vi "Actor.vi"(0 "Path":path, 4 "Creator":refnum<user-event>, 6 "Creator Alias":string, 8 "Self Alias":string, 9 "Queue of Created Info":refnum<queue>, 10 "Actor":refnum<class "Actor.lvclass">) -> ()   [LabVIEW 2021, in "jettl.lvlib" / "Actor.lvlib" / "Base Actor.lvclass"]
uses:
  Base Actor.lvclass
  Actor/Actor.lvclass
  Msg/Msg.lvclass
  Created Info/Created Info.lvclass
  C:/git/jettl/jettl/jettl/Actor/Actor/Actor.lvclass
  Base Actor.lvclass/Base Actor.ctl
  Addresses Strategy/Addresses Strategy.lvlib
  Last Ack Msg/Last Ack Msg.lvlib
  C:/git/jettl/jettl/jettl/Last Ack Msg/Last Ack/Last Ack.lvclass
  C:/git/jettl/jettl/jettl/Setup Msg/Setup/Setup.lvclass
  C:/git/jettl/jettl/jettl/Teardown Msg/Teardown/Teardown.lvclass
  Actor.lvlib
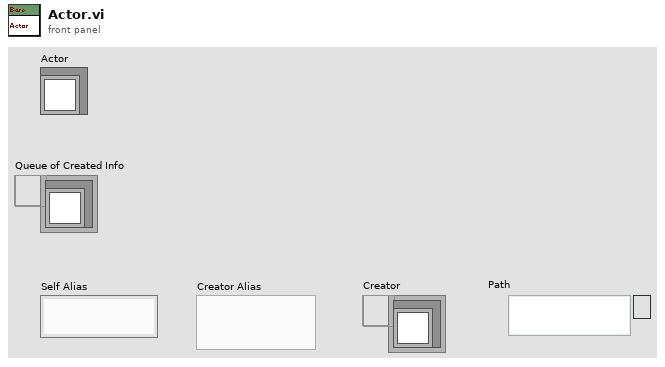
[diagram p1: front panel]
types:
  T1 = typedef "jettl.lvlib/Utilities.lvlib/Set of Msgs.ctl" = set{refnum<class "Msg.lvclass">}
  T2 = typedef "jettl.lvlib/Utilities.lvlib/Created Aliases.ctl" = set{string}
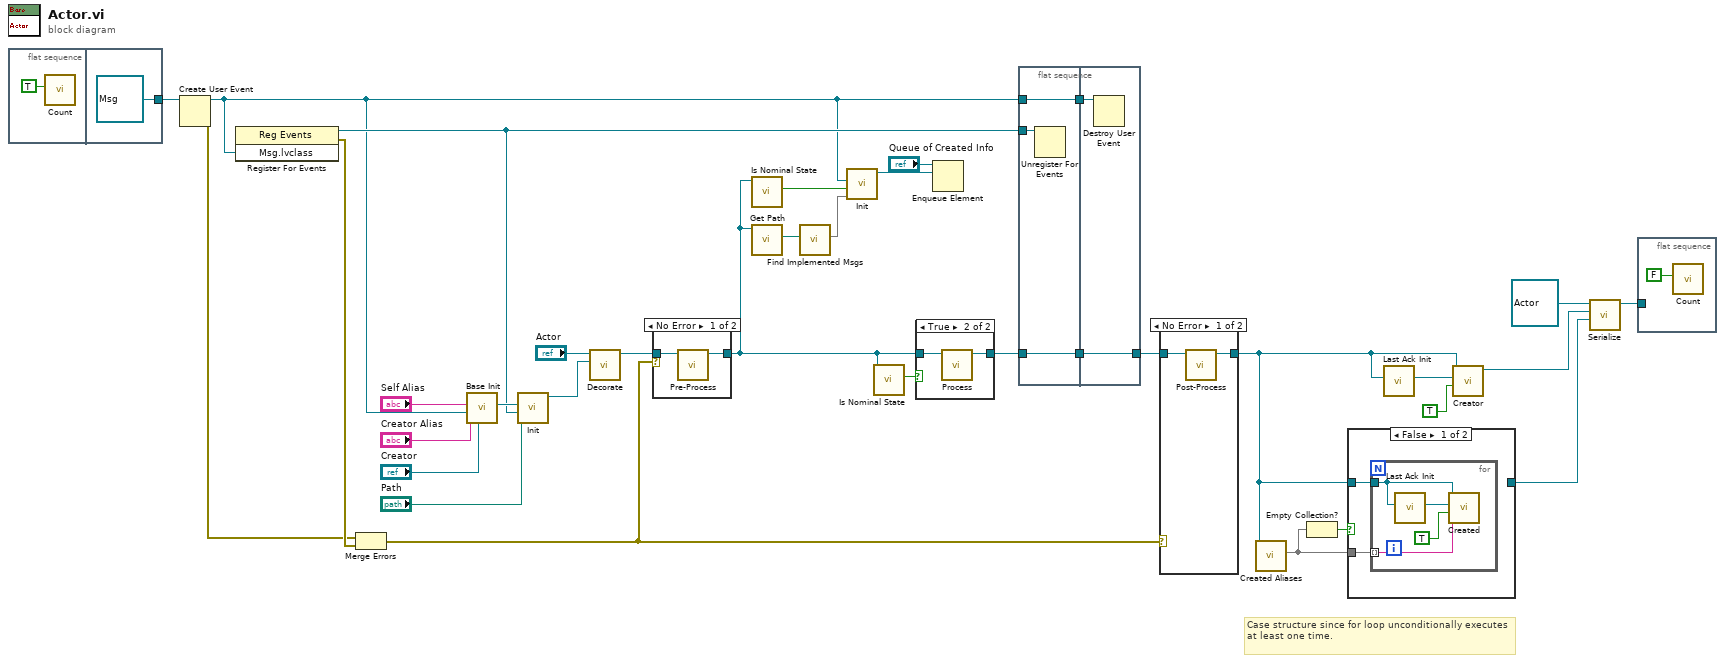
[diagram p0: block diagram]
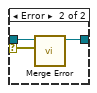
[diagram p2: hidden frame]
diagram:
  # "Case structure since for loop unconditionally executes at least one time."
  n1 = flat-sequence {
    tunnel: [refnum<class "Msg.lvclass"> refnum ("Msg.lvclass")] -> w28
    frame #0 {
      n2 = call "Count.vi"("Increment?"=TRUE) -> ()  [unwired: 11 in]
    }
    frame #1 {
    }
  }
  n3 = Create User Event(user event datatype=w28) -> (user event=w6:refnum<user-event>, error out=w30:errorcluster)  [unwired: 1 in]
  n4 = register-events(w6) -> (reference out=w21:refnum<event-registration>, error out=w32:errorcluster)  [unwired: 2 in]
  n5 = Merge Errors(w30, w32) -> (w18:errorcluster)
  n6 = call "Base Init.vi"("Creator"="Creator", "Creator Alias"="Creator Alias", "Self"=w6, "Self Alias"="Self Alias") -> ("Addresses Strategy out"=w29:refnum<class "Addresses Strategy.lvclass">)  [unwired: 7 in]
  n7 = call "Init.vi"("Path"="Path", "Register"=w21, "Addresses Strategy"=w29) -> ("Base Actor out"=w26:refnum<class "Base Actor.lvclass">)  [unwired: 8 in]
  n8 = call-dynamic "Decorate.vi"("Actor"=w26, "Actor in"="Actor") -> ("Actor out"=w25:refnum<class "Actor.lvclass">)  [unwired: 9 in]
  n9 = case shown="No Error" w18 {
    selector: w18 -> [_ w39]
    tunnel: [w38 w40] -> w3
    tunnel: w25 -> [w37 w41]
    frame No Error {
      n10 = call-dynamic "Pre-Process.vi"("Actor in"=w37) -> ("Actor out"=w38:refnum<class "Actor.lvclass">)  [unwired: 10 in]
    }
    frame Error {
      n11 = call-dynamic "Merge Error.vi"("Error"=w39, "Actor in"=w41) -> ("Actor out"=w40:refnum<class "Actor.lvclass">)  [unwired: 9 in]
    }
  }
  n12 = call-dynamic "Is Nominal State.vi"("Actor in"=w3) -> ("Is Nominal State?"=w2:bool)  [unwired: 10 in]
  n13 = call-dynamic "Get Path.vi"("Actor in"=w3) -> ("Path"=w4:path)  [unwired: 10 in]
  n14 = call "Find Implemented Msgs.vi"("Path"=w4) -> ("Set of Msgs"=w5:T1)  [unwired: 10 in]
  n15 = call "Init.vi"("Set of Msgs"=w5, "Is Normal"=w2, "Self"=w6) -> ("Created Info out"=w7:refnum<class "Created Info.lvclass">)  [unwired: 8 in]
  n16 = call-dynamic "Is Nominal State.vi"("Actor in"=w3) -> ("Is Nominal State?"=w1:bool)  [unwired: 10 in]
  n17 = case shown="True" w1 {
    tunnel: w3 -> [w42 w44]
    tunnel: [w42 w43] -> w22
    frame False {
    }
    frame True {
      n18 = call-dynamic "Process.vi"("Actor in"=w44) -> ("Actor out"=w43:refnum<class "Actor.lvclass">)  [unwired: 10 in]
    }
  }
  n19 = Enqueue Element(queue="Queue of Created Info", element=w7) -> ()  [unwired: 2 in, 3 out]
  n20 = flat-sequence {
    tunnel: [w47] -> w23
    tunnel: w22 -> [w47]
    tunnel: w21 -> [w46]
    tunnel: w6 -> [w45]
    tunnel: [w45] -> w20
    tunnel: [w49] -> w24
    tunnel: w23 -> [w49]
    tunnel: w20 -> [w48]
    frame #0 {
      n21 = Unregister For Events(event registration refnum=w46) -> ()  [unwired: 1 in, 1 out]
    }
    frame #1 {
      n22 = Destroy User Event(user event=w48) -> ()  [unwired: 1 in, 1 out]
    }
  }
  n23 = case shown="No Error" w18 {
    tunnel: w24 -> [w51 w52]
    tunnel: [w50 w52] -> w12
    frame No Error {
      n24 = call-dynamic "Post-Process.vi"("Actor in"=w51) -> ("Actor out"=w50:refnum<class "Actor.lvclass">)  [unwired: 10 in]
    }
    frame Error {
    }
  }
  n25 = call-dynamic "Created Aliases.vi"("Actor in"=w12) -> ("Created Aliases"=w14:T2)  [unwired: 10 in]
  n26 = Empty Collection?(1:w14) -> (0:w15:bool)
  n27 = case shown="False" w15 {
    tunnel: w14 -> [w54 _]
    tunnel: w12 -> [w53 w59]
    tunnel: [_ w59] -> w10
    frame False {
      n28 = for {
        tunnel: w53 -> [w56]
        tunnel: w54 -> [w58] mode=indexing
        n29 = call "Last Ack Init.vi"("Actor"=w56) -> ("Msg"=w55:refnum<class "Msg.lvclass">)  [unwired: 10 in]
        n30 = call-dynamic "Created.vi"("Created Alias"=w58, "Is Priority"=TRUE ("Priority?"), "Msg"=w55, "Actor in"=w56) -> ()  [unwired: 7 in, 1 out]
      }
    }
    frame True {
    }
  }
  n31 = call "Last Ack Init.vi"("Actor"=w12) -> ("Msg"=w16:refnum<class "Msg.lvclass">)  [unwired: 10 in]
  n32 = call-dynamic "Creator.vi"("Is Priority"=TRUE ("Priority?"), "Msg"=w16, "Actor in"=w12) -> ("Actor out"=w11:refnum<class "Actor.lvclass">)  [unwired: 8 in]
  n33 = call-dynamic "Serialize.vi"("Input 2"=w10, "Input 1"=w11, "Actor in"=refnum<class "Actor.lvclass"> refnum ("jettl in")) -> ("Actor out"=w13:refnum<class "Actor.lvclass">)  [unwired: 8 in]
  n34 = flat-sequence {
    tunnel: w13 -> [_]
    frame #0 {
      n35 = call "Count.vi"("Increment?"=FALSE) -> ()  [unwired: 11 in]
    }
  }
